vi "Constants.vi"() -> ()   [LabVIEW 2020, in "FPGA Addon Shared.lvlib"]
doc: "Use this Global VI to access the GUIDs assigned to the page resources of the Custom Device."
uses:
  FPGA Addon Shared.lvlib
panel:
  in  "Tab Control":enum32{"GUIDS", "Constants", "Properties"}(tab)=enum."Constants"
  in  "Group Output":string="58901a15-a42e-477a-af06-3ceeb84f52de"
  in  "Group Input":string="88748f7d-ce11-4328-8f35-56fd574a40c1"
  in  "Speciality IO":string="25832021-24b6-475a-aa84-f4ed7870ed99"
  in  "Static Scalar Output":string="ddc5186b-4b14-4629-b48a-cef4575f789c"
  in  "Static Scalar Input":string="7579cb69-d559-4b2b-a1fc-0d112e8661b6"
  in  "Bitpacked Output":string="6db3f02b-654f-4ed6-bd84-80bb5242a557"
  in  "Bitpacked Input":string="4b03cffd-e469-431a-ba96-aca85ece66af"
  in  "Scalar Output Bitpacked":string="ebfc3e29-7579-49df-b828-0da2c3787b5f"
  in  "Scalar Input Bitpacked":string="8489bf21-57e3-4e68-bdd5-eadff573ec1e"
  in  "FPGA Addon Disabled":string="1903f8c0-e426-4f25-b8ca-65973b1160fd"
  in  "DMA Status Section":string="4e1a084b-2b8b-4128-8417-f0007d9ffe93"
  in  "DMA Channel":string="fdfaa619-d09f-452b-8143-c1a261c13b7a"
  in  "DMA Elements Remaining":string="785497d1-fc1e-46c9-8feb-aa61f2850cff"
  in  "DMA Error":string="708ff167-b4eb-405e-bb0f-5c2fb305da21"
  in  "Waveform Status":string="7b14568c-1c57-4b29-927d-b868126174e2"
  in  "Waveform Input":string="2afc1de4-b056-47bb-a2ad-eec5ad0d30b6"
  in  "Waveform Output":string="0c0ecc88-7768-47db-a589-856e32a93156"
  in  "Waveform Outputs":string="bc66db3e-ace6-4d58-add4-89e89e885df7"
  in  "Scalar Output":string="625afbbf-e929-46eb-93d1-fe7033ba1e7b"
  in  "Scalar Input":string="9bd0c044-925c-4d1d-a44e-de3c4043858c"
  in  "Waveform Inputs":string="165959cb-b691-43bd-9f8b-54fe62f4b534"
  in  "Waveforms":string="5f75895a-bfdb-4cd8-9ef2-787e261eba38"
  in  "Scalar Outputs":string="7d46fed9-731a-4423-8f13-aa8ac2cd791c"
  in  "Scalar Inputs":string="45f50bc5-dab3-4e15-b99b-0f8c8c0fe0f0"
  in  "Scalars":string="884b7050-623e-4f2c-925b-6b753ddf9d1a"
  in  "FPGA Addon":string="e80a28c5-621d-4211-b584-b71df509dee0"
  in  "WFM_OFFSET":string="offset from start"
  in  "WFM_DT":string="dt"
  in  "WFM_T0":string="t0 at start"
  in  "Help.FileName":string="FPGA Addon.chm"
  out "DMA Error Codes":cluster{"number":i32, "trimmed string":string}[](array[cluster])=[{"number"=0, "trimmed string"="<0> No Error."}, {"number"=-61219, "trimmed string"="<-61219> The number of elements requested must be less than or equal to the number of unacquired elements left in the host memory DMA FIFO."}, {"number"=-61217, "trimmed string"="<-61217> A session cannot be closed or reset and a bitfile cannot be downloaded while DMA FIFO region references are outstanding for the specified session."}, {"number"=-61082, "trimmed string"="<-61082> The current target does not have sufficient DMA control line sets available."}, {"number"=-61081, "trimmed string"="<-61081> Insufficient DMA channels available on the current target."}, {"number"=-61077, "trimmed string"="<-61077> Terminated DMA FIFO."}, {"number"=-61076, "trimmed string"="<-61076> The DMA transfer did not complete within the timeout period."}, {"number"=-61075, "trimmed string"="<-61075> The DMA transfer was aborted and did not complete."}, {"number"=-61073, "trimmed string"="<-61073> The number of elements to read or write must be less than or equal to the depth of the host memory DMA FIFO."}, {"number"=-61071, "trimmed string"="<-61071> The selected DMA FIFO was not found in the bitfile or FPGA design or is out of sync with the bitfile."}, {"number"=-61053, "trimmed string"="<-61053> Insufficient DMA channels available."}, {"number"=-61051, "trimmed string"="<-61051> Multiple FIFOs using the same DMA channel."}, {"number"=-61048, "trimmed string"="<-61048> This target does not support DMA output from the host to the target."}]
  in  "Source WFM":string="Source WFM"
  in  "DMA Status Section Name":string="Status Channels"
  in  "Object Not Added Text":string="- Not Added -"
  in  "Bitfile Object Name":string="Bitfile Object Name"
  in  "Bitfile":string="Bitfile"
  in  "Available DMA":string="Available DMA"
  in  "Available Registers":string="Available Registers"
  in  "FPGA Addon Name":string="FPGA Addon"
  in  "Scalars Name":string="Scalars"
  in  "Scalar Inputs Name":string="Scalar Inputs"
  in  "Scalar Outputs Name":string="Scalar Outputs"
  in  "Waveforms Name":string="Waveforms"
  in  "Waveform Inputs Name":string="Waveform Inputs"
  in  "Scalar Input Name":string="Scalar Input"
  in  "Scalar Output Name":string="Scalar Output"
  in  "Waveform Outputs Name":string="Waveform Outputs"
  in  "Waveform Output Name":string="Waveform Output"
  in  "Waveform Input Name":string="Waveform Input"
  in  "Waveform Status Name":string="Waveform Status"
  in  "DMA Error Name":string="Error Code"
  in  "DMA Elements Remaining Name":string="Elements Remaining"
  in  "FPGA.Group":string="Group"
  in  "DMA.HostBuffer":string="DMA.HostBuffer"
  in  "DMA.NumberOfSamples":string="DMA.NumberOfSamples"
  in  "DMA.Mode":string="DMA.Mode"
  in  "Settings.Compiled":string="Settings.Compiled"
  in  "DMA.dt":string="DMA.dt"
  in  "DMA.UpdateRate":string="DMA.UpdateRate"
  in  "DMA.DelacingScheme":string="DMA.DelacingScheme"
  in  "DMA.NumberOfChans":string="DMA.NumberOfChans"
  in  "FPGA.Device":string="FPGA.Device"
  in  "FPGA.Bitfile":string="FPGA.Bitfile"
  in  "Scalar.NumberOfChans":string="Scalar.NumberOfChans"
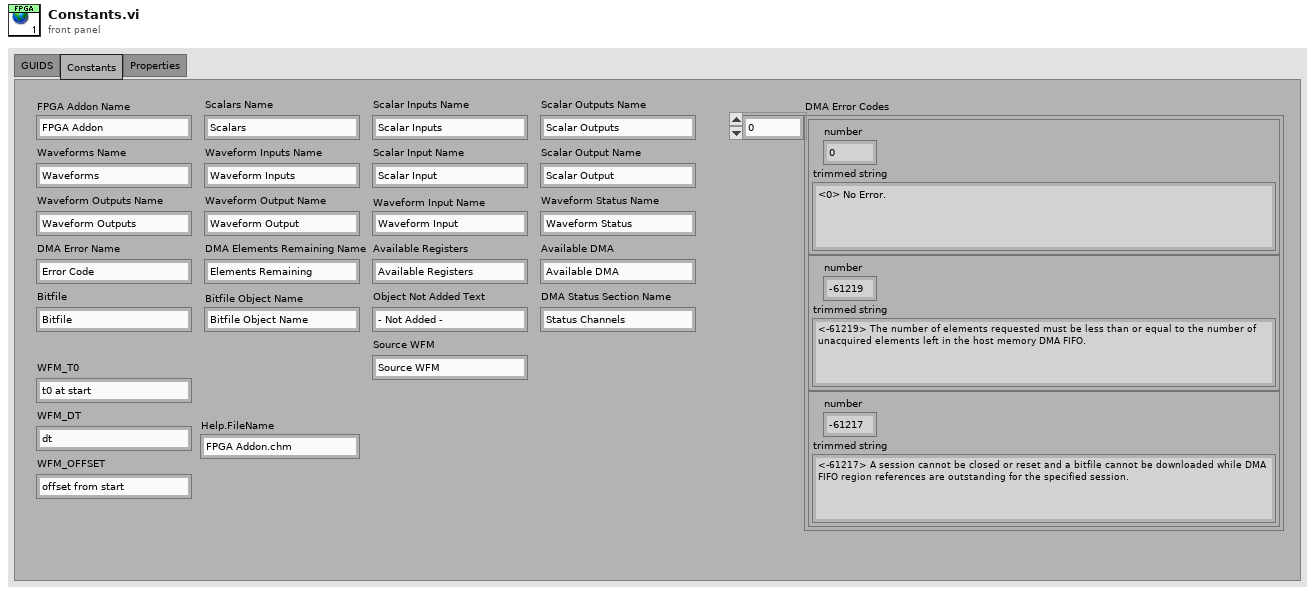
[diagram p1: front panel]
diagram:
